vi "SubVi_Activar.vi"(9 "Indice de Alarma":i32, 10 "Nombre de Alarma":string="Pánico", 11 "input cluster":T1) -> (3 "output cluster":T1)   [LabVIEW 2017]
uses:
  Cluster_Inicial.ctl
  <vilib>/Modbus/master/Modbus Master.lvclass
  <vilib>/addons/_office/excel.llb/Excel Get Data (dbl).vi
  <vilib>/addons/_office/excel.llb/Excel Easy Table (str).vi
  <vilib>/Utility/NIReport.llb/NI_report.lvclass
  <vilib>/addons/_office/NI_ReportGenerationToolkit.lvlib
  <vilib>/Utility/NIReport.llb/Excel/NI_Excel.lvclass
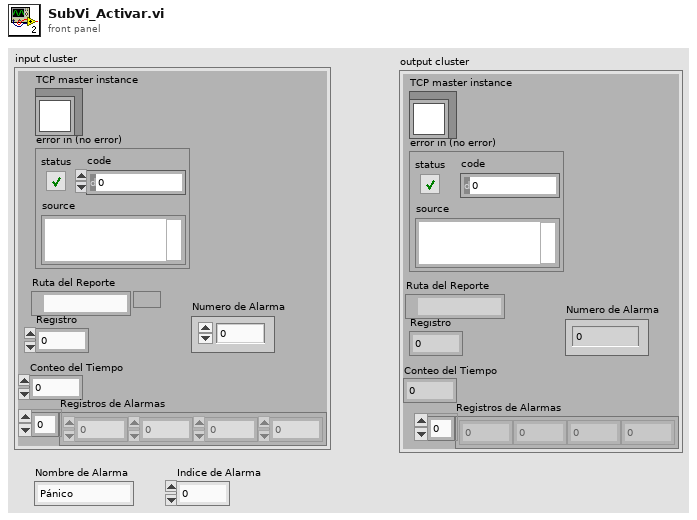
[diagram p1: front panel]
types:
  T1 = typedef "Cluster_Inicial.ctl" = cluster{"TCP master instance":refnum<class "Modbus Master.lvclass">, "error in (no error)":errorcluster, "Ruta del Reporte":path, "Registro":i32, "Conteo del Tiempo":i32, "Registros de Alarmas":i32[], "Numero de Alarma":u32}
  T2 = enum16{"maximized", "minimized", "normal", "no change"}
  T3 = enum16{"Standard Report", "HTML", "Word", "Excel"}
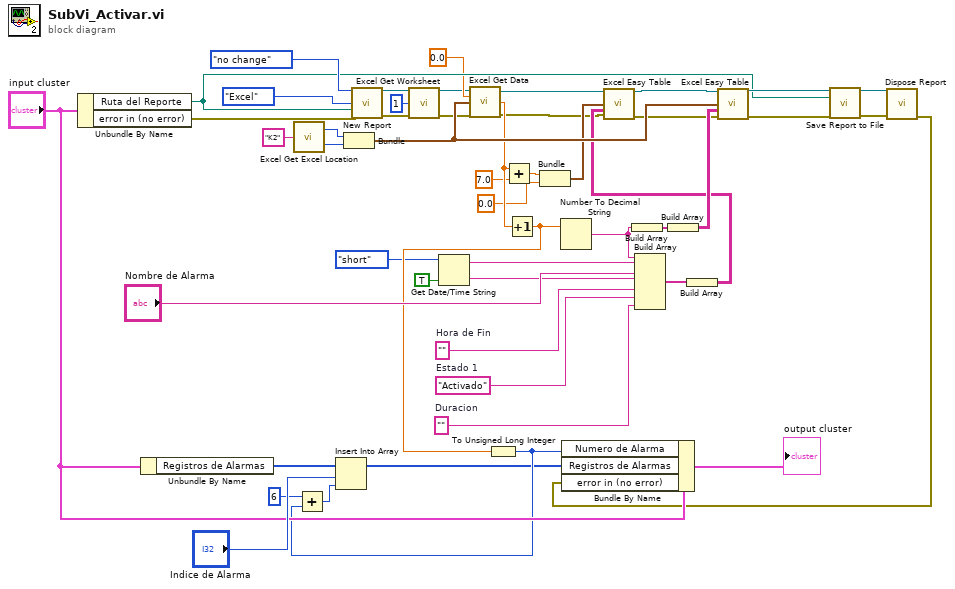
[diagram p0: block diagram]
diagram:
  w9 = ""  # Duracion
  w12 = "Activado"  # Estado 1
  w15 = ""  # Hora de Fin
  n1 = Unbundle By Name("input cluster") -> ("Ruta del Reporte"=w37:path, "error in (no error)"=w29:errorcluster)
  n2 = Unbundle By Name("input cluster") -> ("Registros de Alarmas"=w14:i32[])
  n3 = call <vilib>:"Excel Get Excel Location.vi"("cell's name"="K2") -> ("row"=w27:i32, "column"=w28:i32)
  n4 = Bundle("row"=w27, "column"=w28) -> (w46:cluster{"row":i32, "column":i32})  [unwired: 1 in]
  n5 = call <vilib>:"New Report.vi"("window state (normal)"=T2."no change", "report type"=T3."Excel", "template (empty)"=w37, "error in (no error)"=w29) -> ("report out"=w22:refnum<class "NI_report.lvclass">, "error out"=w23:errorcluster)  [unwired: 10 in]
  n6 = call <vilib>:"Excel Get Worksheet.vi"("report in"=w22, "worksheet index (0)"=1, "error in (no error)"=w23) -> ("report out"=w21:refnum<class "NI_report.lvclass">, "error out"=w20:errorcluster)  [unwired: 11 in]
  n7 = Get Date/Time String(date format (0)=enum16{"short", "long", "abbreviated"}."short", want seconds? (F)=TRUE) -> (date string=w41:string, time string=w16:string)  [unwired: 1 in]
  n8 = call-poly <vilib>:"Excel Get Data.vi"("report in"=w21, "data type"=0.0, "start (0, 0)"=w46, "error in (no error)"=w20) -> ("report out"=w18:refnum<class "NI_report.lvclass">, "data"=w38:dbl, "error out"=w19:errorcluster)  [unwired: 9 in]
  n9 = Add(x=w38, y=7.0) -> (x+y=w32:dbl)
  n10 = Increment(x=w38) -> (x+1=w11:dbl)
  n11 = To Unsigned Long Integer(number=w11) -> (unsigned 32bit integer=w5:u32)
  n12 = Add(x=u32 6, y=w5) -> (x+y=w6:u32)
  n13 = Insert Into Array(array=w14, index="Indice de Alarma", new element=w6) -> (w3:i32[])
  n14 = Bundle(w32, 0.0) -> (w34:cluster{dbl, dbl})  [unwired: 1 in]
  n15 = Number To Decimal String(number=w11) -> (decimal integer string=w47:string)  [unwired: 1 in]
  n16 = Build Array(w47) -> (w48:string[])
  n17 = Build Array(w47, w41, "Nombre de Alarma", w16, w15, w12, w9) -> (w39:string[])
  n18 = Build Array(w48) -> (w49:string[][])
  n19 = Build Array(w39) -> (w40:string[][])
  n20 = call-poly <vilib>:"Excel Easy Table.vi"("report in"=w18, "start (0, 0)"=w34, "text data"=w40, "error in (no error)"=w19) -> ("report out"=w43:refnum<class "NI_report.lvclass">, "error out"=w44:errorcluster)  [unwired: 7 in, 3 out]
  n21 = call-poly <vilib>:"Excel Easy Table.vi"("report in"=w43, "start (0, 0)"=w46, "text data"=w49, "error in (no error)"=w44) -> ("report out"=w50:refnum<class "NI_report.lvclass">, "error out"=w45:errorcluster)  [unwired: 7 in, 3 out]
  n22 = call-dynamic "Save Report to File.vi"("report in"=w50, "report file path"=w37, "error in (no error)"=w45) -> ("report out"=w35:refnum<class "NI_report.lvclass">, "error out"=w36:errorcluster)  [unwired: 11 in]
  n23 = call-dynamic "Dispose Report.vi"("report in"=w35, "error in (no error)"=w36) -> ("error out"=w7:errorcluster)  [unwired: 13 in]
  n24 = Bundle By Name(cluster="input cluster", "Numero de Alarma"=w5, "Registros de Alarmas"=w3, "error in (no error)"=w7) -> (→"output cluster":T1)
